vi "Loop.vi"(8 "error in":errorcluster, 10 "UI Queue":refnum<queue>, 11 "Listener Queue":T1) -> (0 "error out":errorcluster)   [LabVIEW 2019, in "Listener.lvlib"]
uses:
  Listener.lvlib
  Listener Message Queue.ctl
  Listener Message.ctl
  Listener Command.ctl
  UI/Update Message.ctl
  UI/Update Command.ctl
  Listener States.ctl
  Controller/Serial Info.ctl
  Controller/Controller States.ctl
  <vilib>/Instr/_visa.llb/Select Event Type.ctl
  <vilib>/Instr/_visa.llb/VISA Configure Serial Port (Instr).vi
  Controller/Controller.lvlib
  UI/UI.lvlib
panel:
  out "TEMP RESULT":string[](array[string])
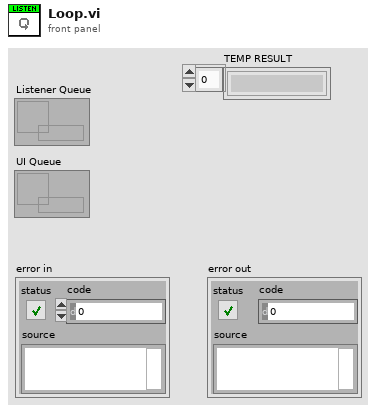
[diagram p1: front panel]
types:
  T1 = typedef "Listener.lvlib/Listener Message Queue.ctl" = refnum<queue>
  T2 = typedef "Listener.lvlib/Listener Message.ctl" = cluster{"Listener Command":T3, "Value":variant}
  T3 = typedef "Listener.lvlib/Listener Command.ctl" = enum16{"Idle", "Open", "Incoming", "Close", "Error", "Stop"}
  T4 = typedef "Listener.lvlib/Listener States.ctl" = cluster{"Resource":refnum<visa-resource-name>}
  T5 = typedef "Controller.lvlib/Controller States.ctl" = cluster{"Resource":refnum<visa-resource-name>}
  T6 = typedef "Controller.lvlib/Serial Info.ctl" = cluster{"Port":refnum<visa-resource-name>, "Baud Rate":u32}
  T7 = typedef "Select Event Type.ctl" = u32
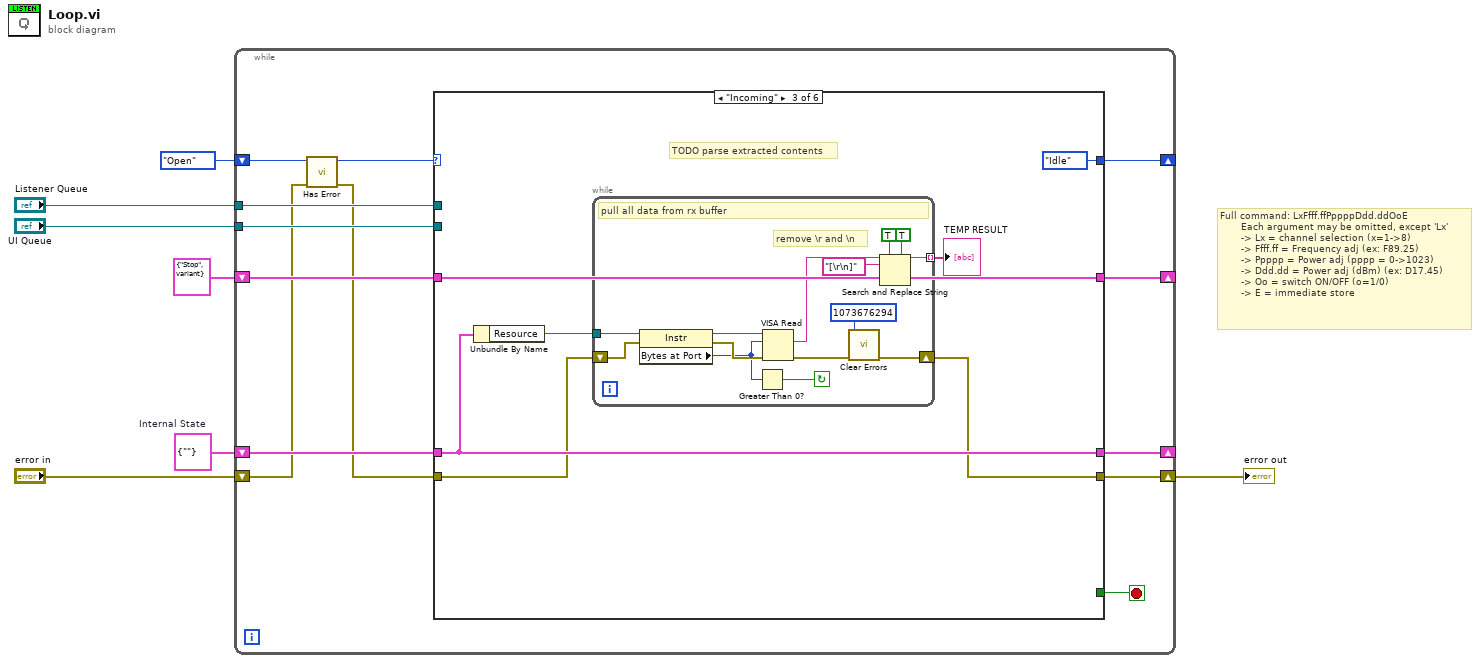
[diagram p0: block diagram]
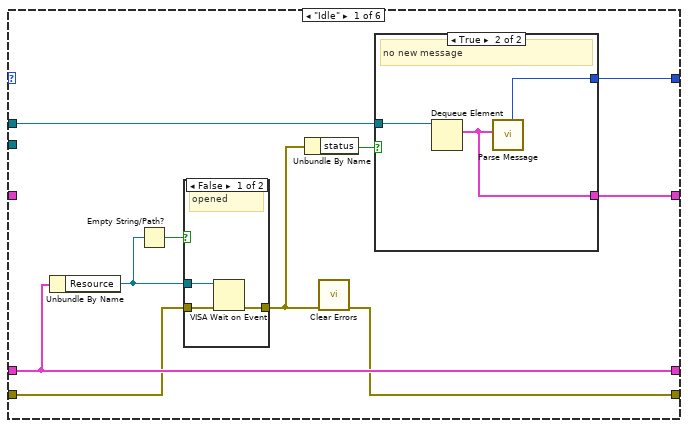
[diagram p2: hidden frame]
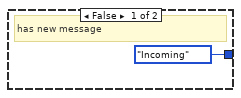
[diagram p3: hidden frame]
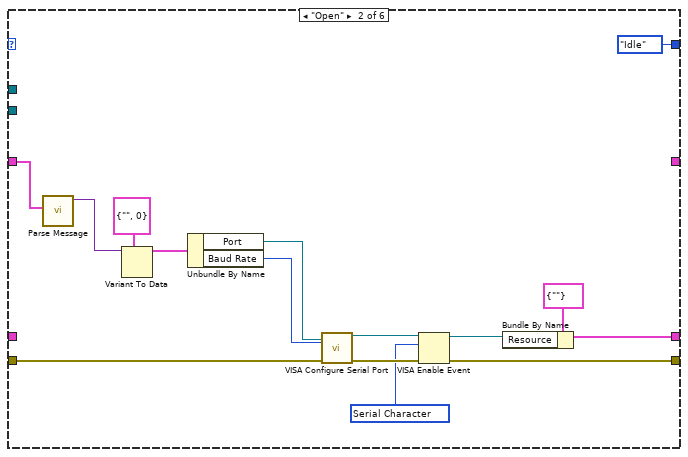
[diagram p5: hidden frame]
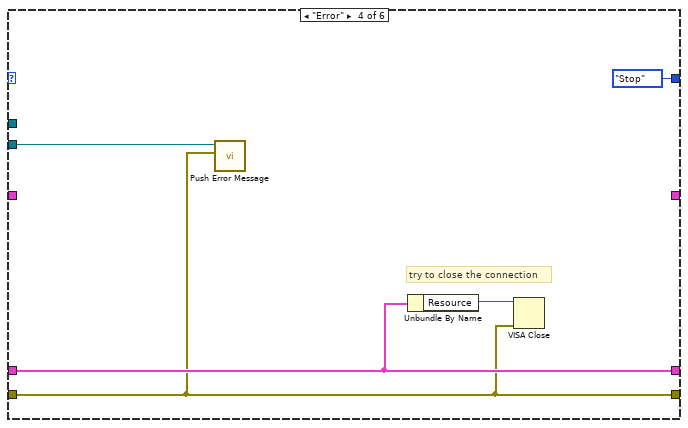
[diagram p6: hidden frame]
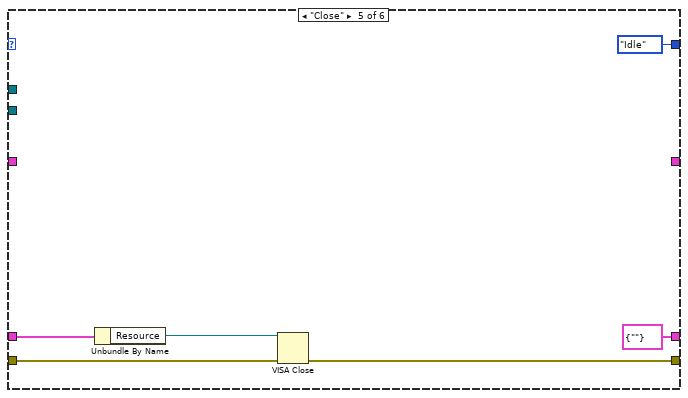
[diagram p7: hidden frame]
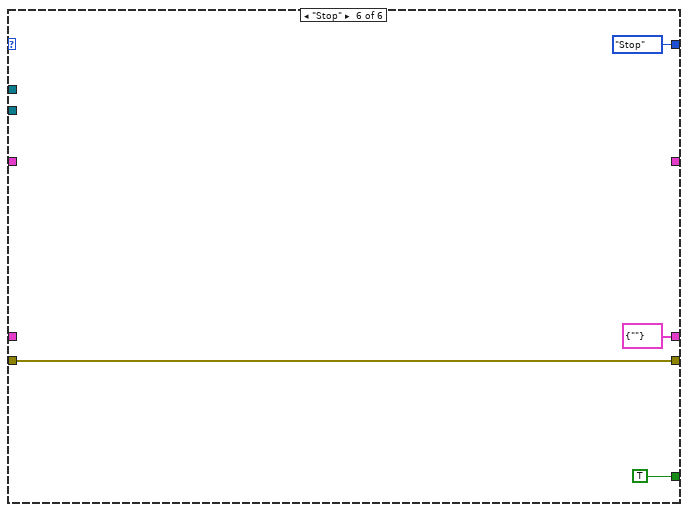
[diagram p8: hidden frame]
diagram:
  w7 = T4 {"Resource"=""}  # Internal State
  # "Full command: LxFfff.ffPppppDdd.ddOoE\n       Each argument may be omitted, except 'Lx'\n       -> Lx = channel selection (x=1->8)\n       -> Ffff.ff = Frequency adj (ex: F89.25)\n       -> Ppppp = Power adj (pppp = 0->1023)\n       -> Ddd.dd = Power adj (dBm) (ex: D17.45)\n       -> Oo = switch ON/OFF (o=1/0)\n       -> E = immediate store"
  n1 = while {
    tunnel: "Listener Queue" -> [w17]
    shift-right: [w20] -> _
    shift-left: w7 -> [w19]
    shift-right: [w15] -> w5
    shift-left: "error in" -> [w9]
    shift-right: [w8] -> _
    shift-left: T2 {"Listener Command"=enum."Stop", "Value"=variant} ("Listener Message") -> [w16]
    shift-right: [w13] -> _
    shift-left: Listener_Command."Open" ("Listener Command") -> [w12]
    tunnel: "UI Queue" -> [w14]
    stop <- w18 stop-if-true
    # "app listener"
    n2 = call "Has Error.vi"("error in (no error)"=w9, "Listener Command in"=w12) -> ("error out"=w10:errorcluster, "Listener Command out"=w11:T3)  [unwired: 8 in]
    n3 = case shown="\"Incoming\"" w11 {
      tunnel: [w27 w49 w58 w78 T5 {"Resource"=""} T5 {"Resource"=""}] -> w20
      tunnel: w19 -> [w27 _ w58 w78 w84 _]
      tunnel: w10 -> [w24 w47 w56 w75 w82 w89]
      tunnel: [w21 w42 w55 w75 w81 w89] -> w15
      tunnel: [_ _ _ _ _ TRUE] -> w18
      tunnel: w17 -> [w30 _ _ _ _ _]
      tunnel: w16 -> [_ w44 w60 _ _ _]
      tunnel: [w28 Listener_Command."Idle" ("Listener Command") Listener_Command."Idle" ("Listener Command") Listener_Command."Stop" ("Listener Command") Listener_Command."Idle" ("Listener Command") Listener_Command."Stop" ("Listener Command")] -> w13
      tunnel: w14 -> [_ _ _ w76 _ _]
      tunnel: [w29 _ w60 _ _ _] -> w8
      frame "Idle" {
        n4 = Unbundle By Name(w27) -> ("Resource"=w25:refnum<visa-resource-name>)
        n5 = Empty String/Path?(string/path=w25) -> (empty?=w26:bool)
        n6 = case shown="False" w26 {
          tunnel: w25 -> [w37 _]
          tunnel: w24 -> [w36 w38]
          tunnel: [w35 w38] -> w22
          frame False {
            # "opened"
            n7 = VISA Wait on Event(8:w36, 11:w37) -> (0:w35:errorcluster)  [unwired: 3 in, 3 out]
          }
          frame True {
            # "empty path, not opened"
          }
        }
        n8 = Unbundle By Name(w22) -> ("status"=w23:bool)
        n9 = call <vilib>:"Clear Errors.vi"("error in (no error)"=w22) -> ("error out"=w21:errorcluster)  [unwired: 5 in, 1 out]
        n10 = case shown="True" w23 {
          tunnel: w30 -> [_ w34]
          tunnel: [_ w33] -> w29
          tunnel: [Listener_Command."Incoming" ("Listener Command") w32] -> w28
          frame False {
            # "has new message"
          }
          frame True {
            # "no new message"
            n11 = Dequeue Element(queue=w34) -> (element=w33:T2)  [unwired: 2 in, 3 out]
            n12 = call "Parse Message.vi"("Listener Message"=w33) -> ("Listener Command"=w32:T3)  [unwired: 8 in, 1 out]
          }
        }
      }
      frame "Open" {
        w39 = T7 1073684533 items=["Service Request"=1073684491, "Trigger"=3221168138, "Clear"=1073684493, "VXI Signal"=1073684512, "VXI/VME Interrupt"=3221168161, "VXI/VME Sysfail"=1073684509, "VXI/VME Sysreset"=1073684510, "GPIB CIC"=1073684498, "GPIB Talk"=1073684499, "GPIB Listen"=1073684500, "PXI Interrupt"=1073684514, "Serial Break"=1073684515, "Serial TermChar"=1073684516, "Serial CTS"=1073684521, "Serial DSR"=1073684522, "Serial DCD"=1073684524, "Serial RI"=1073684526, "Serial Character"=1073684533, "USB Interrupt"=1073684535, "All Enabled"=1073709055] ("Event Type")
        n13 = call "Parse Message.vi"("Listener Message"=w44) -> ("Value"=w45:variant)  [unwired: 8 in, 1 out]
        n14 = Variant To Data(type=T6 {"Port"="", "Baud Rate"=0} ("Serial Info"), Variant=w45) -> (data=w52:T6)  [unwired: 1 in, 1 out]
        n15 = Unbundle By Name(w52) -> ("Port"=w51:refnum<visa-resource-name>, "Baud Rate"=w50:u32)
        n16 = call-poly "VISA Configure Serial Port"("VISA resource name"=w51, "baud rate (9600)"=w50, "error in (no error)"=w47) -> ("VISA resource name out"=w41:refnum<visa-resource-name>, "error out"=w43:errorcluster)  [unwired: 11 in]
        n17 = VISA Enable Event(8:w43, 10:w39, 11:w41) -> (0:w42:errorcluster, 3:w40:refnum<visa-resource-name>)  [unwired: 1 in]
        n18 = Bundle By Name(cluster=T5 {"Resource"=""}, "Resource"=w40) -> (w49:T5)
      }
      frame "Incoming" {
        # "TODO parse extracted contents"
        n19 = Unbundle By Name(w58) -> ("Resource"=w57:refnum<visa-resource-name>)
        n20 = while {
          tunnel: w57 -> [w74]
          shift-right: [w67] -> w55
          shift-left: w56 -> [w72]
          tunnel: [w61] -> w54 mode=indexing
          stop <- w68 continue-if-true
          # "remove \\r and \\n"
          # "pull all data from rx buffer"
          n21 = property class="Instr"(reference=w74, error in=w72) -> (reference out=w73:refnum<visa-resource-name>, error out=w71:errorcluster, "Bytes at Port"=w69:u32)
          n22 = Greater Than 0?(x=w69) -> (x > 0?=w68:bool)
          n23 = VISA Read(VISA resource name=w73, byte count=w69, error in (no error)=w71) -> (read buffer=w65:string, error out=w70:errorcluster)  [unwired: 2 out]
          n24 = call <vilib>:"Clear Errors.vi"("error in (no error)"=w70, "specific error code to clear (0: all)"=1073676294 ("Code")) -> ("error out"=w67:errorcluster)  [unwired: 4 in, 1 out]
          n25 = Search and Replace String(replace all?=TRUE ("replace all? (F)"), multiline?=TRUE ("multiline? (F)"), input string=w65, search string="[\r\n]") -> (result string=w61:string)  [unwired: 4 in, 3 out]
        }
        "TEMP RESULT" <- w54
      }
      frame "Error" {
        # "try to close the connection"
        n26 = call "Push Error Message.vi"("error constant"=w75, "UI Queue in"=w76) -> ()  [unwired: 9 in, 1 out]
        n27 = Unbundle By Name(w78) -> ("Resource"=w77:refnum<visa-resource-name>)
        n28 = VISA Close(VISA resource name=w77, error in (no error)=w75) -> ()  [unwired: 1 out]
      }
      frame "Close" {
        n29 = Unbundle By Name(w84) -> ("Resource"=w83:refnum<visa-resource-name>)
        n30 = VISA Close(VISA resource name=w83, error in (no error)=w82) -> (error out=w81:errorcluster)
      }
      frame "Stop" {
      }
    }
  }
  "error out" <- w5
